vi "get target by index.vi"(8 "error in":errorcluster, 10 "index":i32, 11 "system hierarchy":T1) -> (0 "error out":errorcluster, 3 "target hierarchy":T1)   [LabVIEW 2013, in "PL_Serialization Interface.lvlib"]
uses:
  PL_Serialization Interface.lvlib
  <vilib>/NI/Configuration Framework/tree serializer/flat hierarchy.ctl
  <vilib>/NI/Configuration Framework/tree serializer/full hierarchy.ctl
  <vilib>/NI/Configuration Framework/tree serializer/hierarchy element.ctl
  <vilib>/NI/Configuration Framework/tree serializer/instance data.ctl
  <vilib>/NI/Configuration Framework/tree serializer/NISE_CEF_TreeSerializer.lvlib
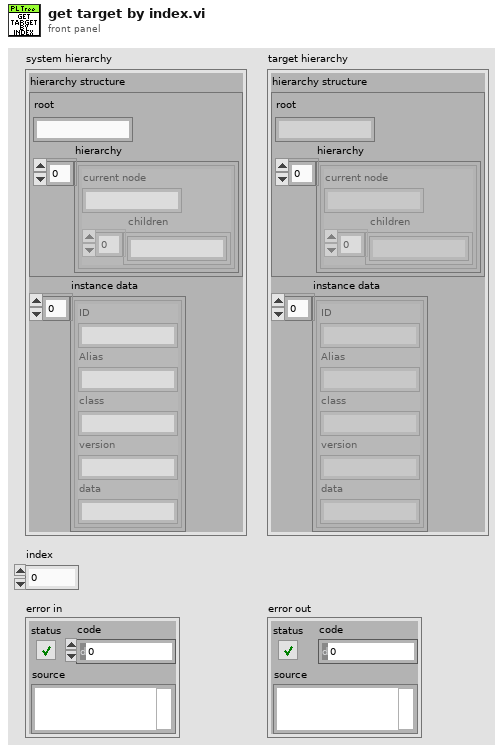
[diagram p1: front panel]
types:
  T1 = typedef "NISE_CEF_TreeSerializer.lvlib/flat hierarchy.ctl" = cluster{"hierarchy structure":T2, "instance data":T4[]}
  T2 = typedef "NISE_CEF_TreeSerializer.lvlib/full hierarchy.ctl" = cluster{"root":string, "hierarchy":T3[]}
  T3 = typedef "NISE_CEF_TreeSerializer.lvlib/hierarchy element.ctl" = cluster{"current node":string, "children":string[]}
  T4 = typedef "NISE_CEF_TreeSerializer.lvlib/instance data.ctl" = cluster{"ID":string, "Alias":string, "class":string, "version":string, "data":string}
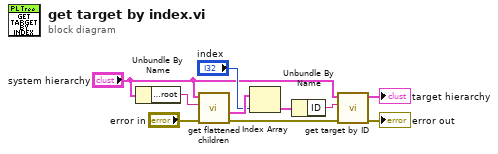
[diagram p0: block diagram]
diagram:
  n1 = Unbundle By Name("system hierarchy") -> ("hierarchy structure.root"=w1:string)
  n2 = call <vilib>:"get flattened children.vi"("error in"="error in", "ID"=w1, "flat hierarchy"="system hierarchy") -> ("error out"=w3:errorcluster, "children"=w6:T4[])  [unwired: 7 in]
  n3 = Index Array(array=w6, index="index") -> (element=w4:T4)
  n4 = Unbundle By Name(w4) -> ("ID"=w9:string)
  n5 = call "get target by ID.vi"("error in"=w3, "UID"=w9, "full system"="system hierarchy") -> ("error out"=→"error out":errorcluster, "target hierarchy"=→"target hierarchy":T1)  [unwired: 7 in]
